vi "Write Coincidences File.vi"(8 "error in (no error)":errorcluster, 11 "Controller in":refnum<class "Controller.lvclass">) -> (0 "error out":errorcluster, 3 "Controller out":refnum<class "Controller.lvclass">)   [LabVIEW 2019, in "Controller.lvlib" / "Controller.lvclass"]
uses:
  Controller.lvclass
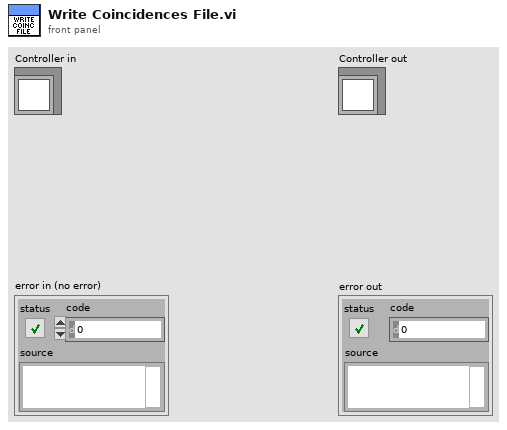
[diagram p1: front panel]
types:
  T1 = typedef "Muon Detector.lvclass/Event.ctl" = cluster{"Event Count":i32, "Device Timestamp (ms)":i32, "PC Timestamp":timestamp, "ADC Count":i32, "Event Type":u8}
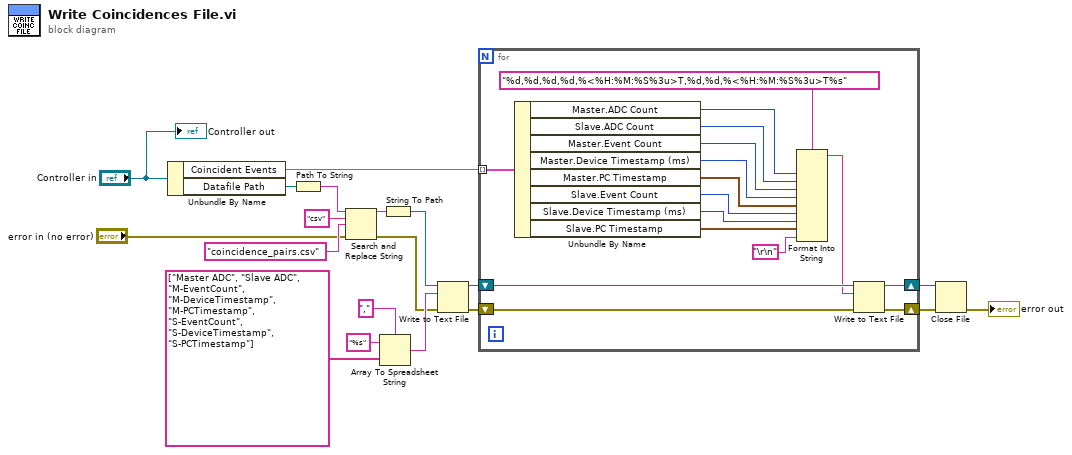
[diagram p0: block diagram]
diagram:
  n1 = Unbundle By Name("Controller in") -> ("Coincident Events"=w11:set{cluster{"Master":T1, "Slave":T1}}, "Datafile Path"=w7:path)
  n2 = Path To String(path=w7) -> (string=w4:string)
  n3 = Search and Replace String(input string=w4, search string="csv" ("substring (\"\")"), replace string="coincidence_pairs.csv" ("replace string (\"\")"), error in="error in (no error)") -> (result string=w8:string, error out=w1:errorcluster)  [unwired: 4 in, 2 out]
  n4 = Array To Spreadsheet String(delimiter (Tab)=",", array=string[] ["Master ADC", "Slave ADC", "M-EventCount", "M-DeviceTimestamp", "M-PCTimestamp", "S-EventCount", "S-DeviceTimestamp", "S-PCTimestamp"], 3:"%s" ("format string")) -> (spreadsheet string=w19:string)
  n5 = String To Path(string=w8) -> (path=w9:path)
  n6 = Write to Text File(file (use dialog)=w9, text=w19, error in=w1) -> (refnum out=w13:refnum<file>, error out=w12:errorcluster)  [unwired: 1 in, 1 out]
  n7 = for {
    tunnel: w11 -> [w35] mode=indexing
    shift-right: [w21] -> w15
    shift-left: w13 -> [w23]
    shift-right: [w22] -> w14
    shift-left: w12 -> [w24]
    n8 = Unbundle By Name(w35) -> ("Master.ADC Count"=w34:i32, "Slave.ADC Count"=w33:i32, "Master.Event Count"=w32:i32, "Master.Device Timestamp (ms)"=w31:i32, "Master.PC Timestamp"=w30:timestamp, "Slave.Event Count"=w29:i32, "Slave.Device Timestamp (ms)"=w28:i32, "Slave.PC Timestamp"=w27:timestamp)
    n9 = Format Into String(format string="%d,%d,%d,%d,%<%H:%M:%S%3u>T,%d,%d,%<%H:%M:%S%3u>T%s", w34, w33, w32, w31, w30, w29, w28, w27, "\r\n") -> (resulting string=w20:string)  [unwired: 2 in, 1 out]
    n10 = Write to Text File(file (use dialog)=w23, text=w20, error in=w24) -> (refnum out=w21:refnum<file>, error out=w22:errorcluster)  [unwired: 1 in, 1 out]
  }
  n11 = Close File(refnum=w15, error in=w14) -> (error out=→"error out":errorcluster)  [unwired: 1 out]
  "Controller out" <- "Controller in"
